vi "Seven-Segment-Display.vi"() -> ()   [LabVIEW 2014]
panel:
  in  "Switch":bool
  in  "stop":bool
  out "e":bool
  out "c":bool
  out "d":bool
  out "f":bool
  out "g":bool
  out "b":bool
  out "a":bool
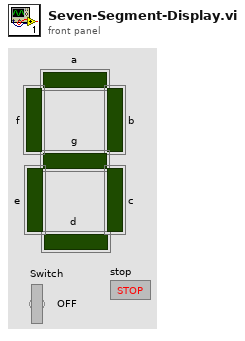
[diagram p1: front panel]
types:
  T1 = enum16{"off", "0", "1", "2", "3", "4", "5", "6", "7", "8", "9"}
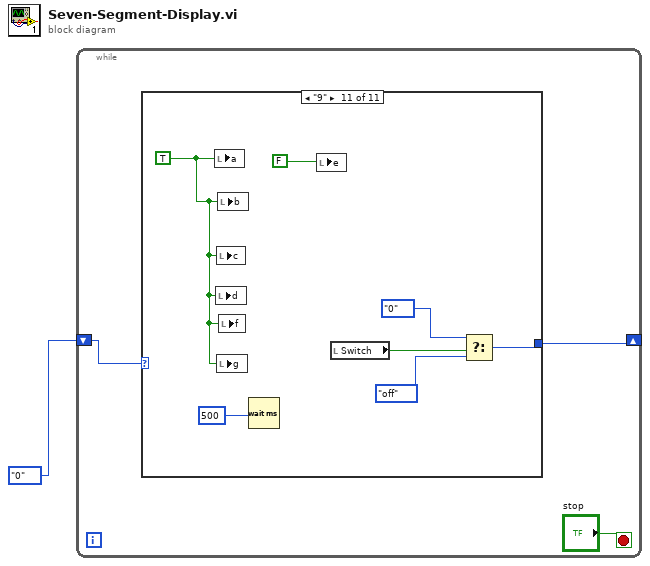
[diagram p0: block diagram]
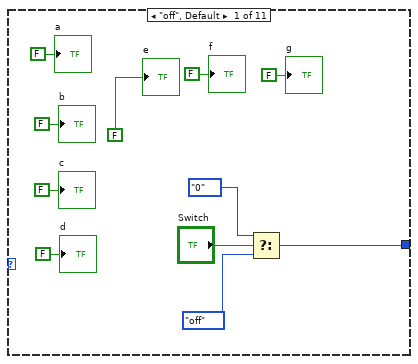
[diagram p2: hidden frame]
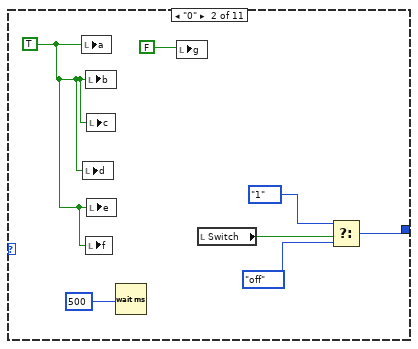
[diagram p3: hidden frame]
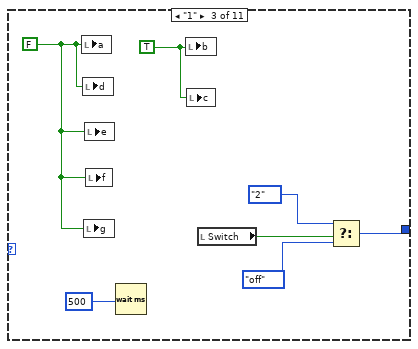
[diagram p4: hidden frame]
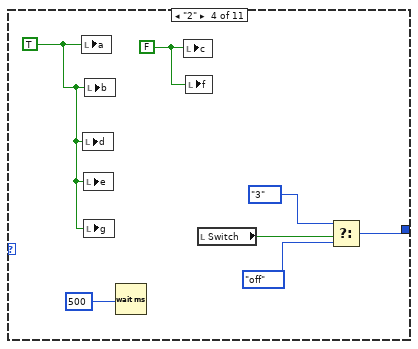
[diagram p5: hidden frame]
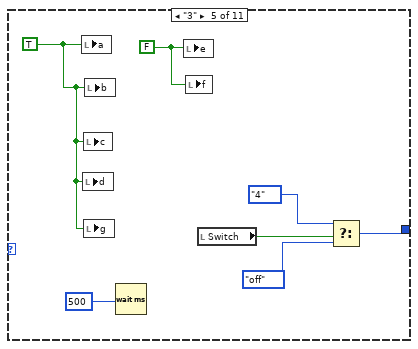
[diagram p6: hidden frame]
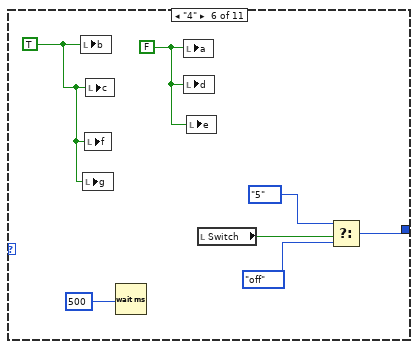
[diagram p7: hidden frame]
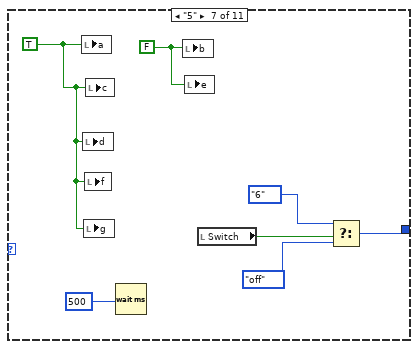
[diagram p8: hidden frame]
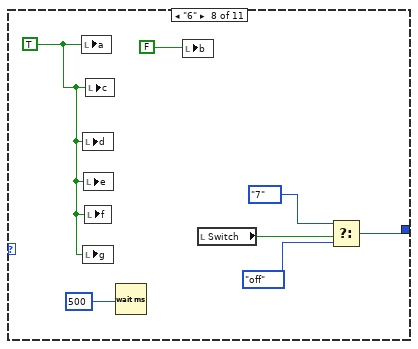
[diagram p9: hidden frame]
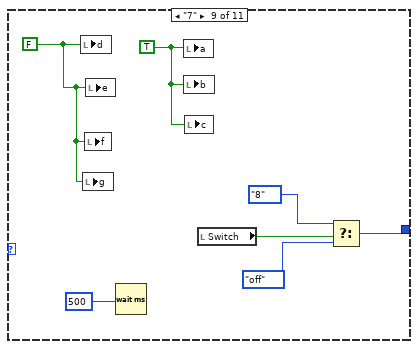
[diagram p10: hidden frame]
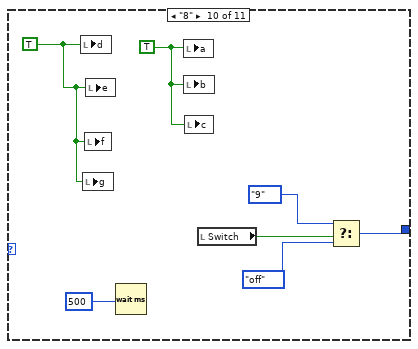
[diagram p11: hidden frame]
diagram:
  n1 = while {
    shift-right: [w2] -> _
    shift-left: T1."0" -> [w3]
    stop <- "stop" stop-if-true
    n2 = case shown="\"9\"" w3 {
      tunnel: [w12 w22 w29 w36 w43 w50 w57 w64 w71 w78 w85] -> w2
      frame "off", Default {
        n3 = Select(t=T1."0", s="Switch", f=T1."off") -> (s? t:f=w12:T1)
        "a" <- FALSE ("a")
        "b" <- FALSE ("b")
        "c" <- FALSE ("c")
        "d" <- FALSE ("d")
        "e" <- FALSE ("e")
        "f" <- FALSE ("f")
        "g" <- FALSE ("g")
      }
      frame "0" {
        w17 = TRUE
        n4 = local write "a"(w17) -> ()
        n5 = local write "d"(w17) -> ()
        n6 = local write "b"(w17) -> ()
        n7 = local write "f"(w17) -> ()
        n8 = local write "c"(w17) -> ()
        n9 = local write "e"(w17) -> ()
        n10 = Wait (ms)(milliseconds to wait=u32 500 ("millisecond timer value")) -> ()  [unwired: 1 out]
        n11 = local write "g"(FALSE) -> ()
        n12 = local read "Switch"() -> (w21:bool)
        n13 = Select(t=T1."1", s=w21, f=T1."off") -> (s? t:f=w22:T1)
      }
      frame "1" {
        w24 = TRUE
        w25 = FALSE
        n14 = local write "a"(w25) -> ()
        n15 = local write "d"(w25) -> ()
        n16 = local write "g"(w25) -> ()
        n17 = local write "e"(w25) -> ()
        n18 = local write "f"(w25) -> ()
        n19 = Wait (ms)(milliseconds to wait=u32 500 ("millisecond timer value")) -> ()  [unwired: 1 out]
        n20 = local write "b"(w24) -> ()
        n21 = local write "c"(w24) -> ()
        n22 = local read "Switch"() -> (w28:bool)
        n23 = Select(t=T1."2", s=w28, f=T1."off") -> (s? t:f=w29:T1)
      }
      frame "2" {
        w30 = FALSE
        w31 = TRUE
        n24 = local write "a"(w31) -> ()
        n25 = local write "d"(w31) -> ()
        n26 = local write "e"(w31) -> ()
        n27 = local write "g"(w31) -> ()
        n28 = local write "b"(w31) -> ()
        n29 = Wait (ms)(milliseconds to wait=u32 500 ("millisecond timer value")) -> ()  [unwired: 1 out]
        n30 = local write "c"(w30) -> ()
        n31 = local write "f"(w30) -> ()
        n32 = local read "Switch"() -> (w35:bool)
        n33 = Select(t=T1."3", s=w35, f=T1."off") -> (s? t:f=w36:T1)
      }
      frame "3" {
        w37 = FALSE
        w38 = TRUE
        n34 = local write "a"(w38) -> ()
        n35 = local write "d"(w38) -> ()
        n36 = local write "c"(w38) -> ()
        n37 = local write "g"(w38) -> ()
        n38 = local write "b"(w38) -> ()
        n39 = Wait (ms)(milliseconds to wait=u32 500 ("millisecond timer value")) -> ()  [unwired: 1 out]
        n40 = local write "e"(w37) -> ()
        n41 = local write "f"(w37) -> ()
        n42 = local read "Switch"() -> (w42:bool)
        n43 = Select(t=T1."4", s=w42, f=T1."off") -> (s? t:f=w43:T1)
      }
      frame "4" {
        w44 = FALSE
        w45 = TRUE
        n44 = local write "b"(w45) -> ()
        n45 = local write "g"(w45) -> ()
        n46 = local write "f"(w45) -> ()
        n47 = local write "c"(w45) -> ()
        n48 = Wait (ms)(milliseconds to wait=u32 500 ("millisecond timer value")) -> ()  [unwired: 1 out]
        n49 = local write "a"(w44) -> ()
        n50 = local write "d"(w44) -> ()
        n51 = local write "e"(w44) -> ()
        n52 = local read "Switch"() -> (w49:bool)
        n53 = Select(t=T1."5", s=w49, f=T1."off") -> (s? t:f=w50:T1)
      }
      frame "5" {
        w51 = FALSE
        w52 = TRUE
        n54 = local write "a"(w52) -> ()
        n55 = local write "d"(w52) -> ()
        n56 = local write "g"(w52) -> ()
        n57 = local write "f"(w52) -> ()
        n58 = local write "c"(w52) -> ()
        n59 = Wait (ms)(milliseconds to wait=u32 500 ("millisecond timer value")) -> ()  [unwired: 1 out]
        n60 = local write "b"(w51) -> ()
        n61 = local write "e"(w51) -> ()
        n62 = local read "Switch"() -> (w56:bool)
        n63 = Select(t=T1."6", s=w56, f=T1."off") -> (s? t:f=w57:T1)
      }
      frame "6" {
        w58 = TRUE
        n64 = local write "a"(w58) -> ()
        n65 = local write "d"(w58) -> ()
        n66 = local write "g"(w58) -> ()
        n67 = local write "e"(w58) -> ()
        n68 = local write "f"(w58) -> ()
        n69 = local write "c"(w58) -> ()
        n70 = Wait (ms)(milliseconds to wait=u32 500 ("millisecond timer value")) -> ()  [unwired: 1 out]
        n71 = local write "b"(FALSE) -> ()
        n72 = local read "Switch"() -> (w63:bool)
        n73 = Select(t=T1."7", s=w63, f=T1."off") -> (s? t:f=w64:T1)
      }
      frame "7" {
        w65 = TRUE
        w66 = FALSE
        n74 = local write "d"(w66) -> ()
        n75 = local write "g"(w66) -> ()
        n76 = local write "f"(w66) -> ()
        n77 = local write "e"(w66) -> ()
        n78 = Wait (ms)(milliseconds to wait=u32 500 ("millisecond timer value")) -> ()  [unwired: 1 out]
        n79 = local write "a"(w65) -> ()
        n80 = local write "b"(w65) -> ()
        n81 = local write "c"(w65) -> ()
        n82 = local read "Switch"() -> (w70:bool)
        n83 = Select(t=T1."8", s=w70, f=T1."off") -> (s? t:f=w71:T1)
      }
      frame "8" {
        w72 = TRUE
        w73 = TRUE
        n84 = local write "d"(w73) -> ()
        n85 = local write "g"(w73) -> ()
        n86 = local write "f"(w73) -> ()
        n87 = local write "e"(w73) -> ()
        n88 = Wait (ms)(milliseconds to wait=u32 500 ("millisecond timer value")) -> ()  [unwired: 1 out]
        n89 = local write "a"(w72) -> ()
        n90 = local write "b"(w72) -> ()
        n91 = local write "c"(w72) -> ()
        n92 = local read "Switch"() -> (w77:bool)
        n93 = Select(t=T1."9", s=w77, f=T1."off") -> (s? t:f=w78:T1)
      }
      frame "9" {
        w79 = TRUE
        n94 = local write "a"(w79) -> ()
        n95 = local write "d"(w79) -> ()
        n96 = local write "c"(w79) -> ()
        n97 = local write "g"(w79) -> ()
        n98 = local write "b"(w79) -> ()
        n99 = local write "f"(w79) -> ()
        n100 = Wait (ms)(milliseconds to wait=u32 500 ("millisecond timer value")) -> ()  [unwired: 1 out]
        n101 = local write "e"(FALSE) -> ()
        n102 = local read "Switch"() -> (w84:bool)
        n103 = Select(t=T1."0", s=w84, f=T1."off") -> (s? t:f=w85:T1)
      }
    }
  }
